vi "Get and Write Data.vi"() -> ()   [LabVIEW 2013]
uses:
  globals_9.vi
panel:
  in  "Количество измерений":u32
  out "Тип измерений":string
  out "Datetime":string
  in  "Operator":string
  in  "Путь к файлу протокола":path
  out "Данные":dbl[](array[numeric])
  in  "Задержка, мс":u32
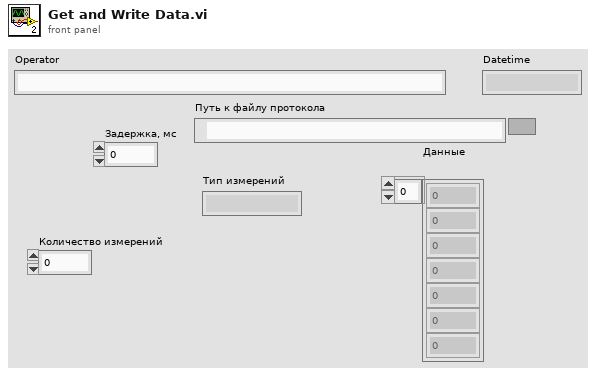
[diagram p1: front panel]
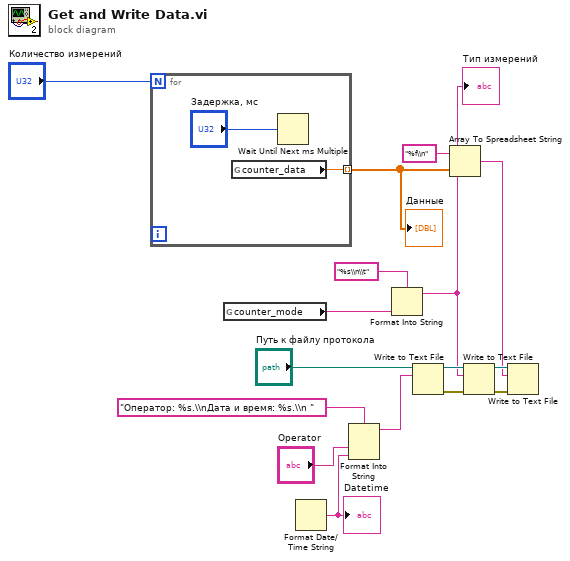
[diagram p0: block diagram]
diagram:
  n1 = for {
    N: "Количество измерений" -> [_]
    tunnel: [w17] -> w5 mode=indexing
    n2 = global read "globals_9.vi" "counter_data"() -> (w17:dbl)
    n3 = Wait Until Next ms Multiple(millisecond multiple="Задержка, мс") -> ()  [unwired: 1 out]
  }
  "Данные" <- w5
  n4 = global read "globals_9.vi" "counter_mode"() -> (w2:string)
  n5 = Format Date/Time String() -> (date/time string=w15:string)  [unwired: 3 in]
  "Datetime" <- w15
  n6 = Format Into String(format string="Оператор: %s.\\nДата и время: %s.\\n ", "Operator", w15) -> (resulting string=w10:string)  [unwired: 2 in, 1 out]
  n7 = Format Into String(format string="%s\\n\\t", w2) -> (resulting string=w3:string)  [unwired: 2 in, 1 out]
  "Тип измерений" <- w3
  n8 = Write to Text File(file (use dialog)="Путь к файлу протокола", text=w10) -> (refnum out=w8:refnum<file>, error out=w13:errorcluster)  [unwired: 2 in, 1 out]
  n9 = Array To Spreadsheet String(array=w5, 3:"%f\\n" ("format string")) -> (spreadsheet string=w6:string)  [unwired: 1 in]
  n10 = Write to Text File(file (use dialog)=w8, text=w3, error in=w13) -> (refnum out=w7:refnum<file>, error out=w12:errorcluster)  [unwired: 1 in, 1 out]
  n11 = Write to Text File(file (use dialog)=w7, text=w6, error in=w12) -> ()  [unwired: 1 in, 3 out]
